vi "Demo_OK_COUNT.vi"(0 "Refnum in":T2, 1 "Station":string, 3 "Shift":i32, 5 "MAX BREAKDOWN ID":i32, 7 "PRODUCTION COUNT":i32, 9 "TABLE NAME":string, 11 "error in (no error)":errorcluster, 12 "Product Code for OK":string) -> (4 "Refnum out":T2, 6 "PROD COUNT":i32, 15 "error out":errorcluster)   [LabVIEW 2017]
uses:
  <vilib>/addons/database/Connection.llb/Conn ObjectReference.ctl
  <vilib>/addons/database/NI_Database_API.lvlib
  <userlib>/_OpenG.lib/comparison/comparison.llb/I32 Changed__ogtk.vi
panel:
  out "output":T1
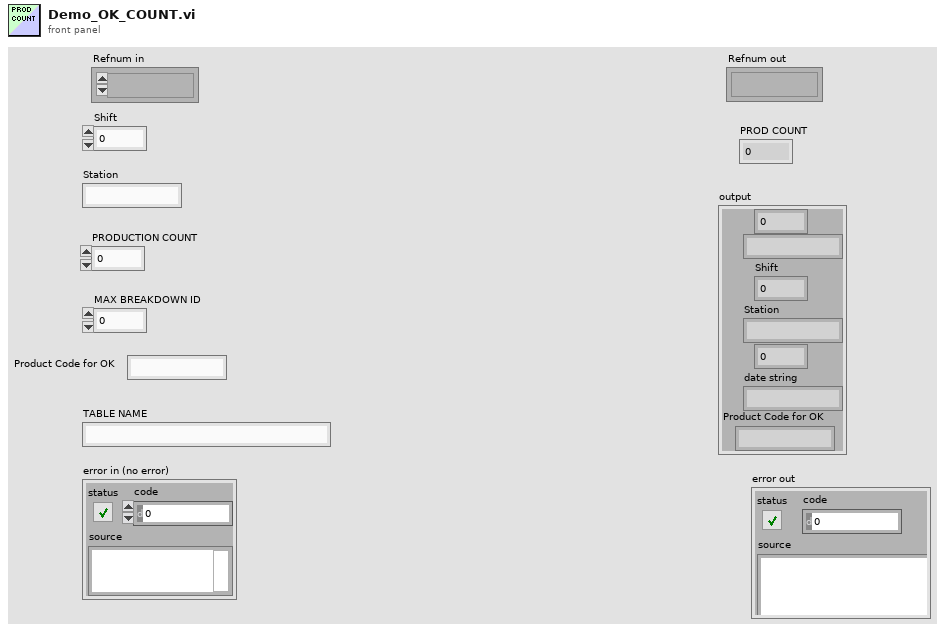
[diagram p1: front panel]
types:
  T1 = cluster{i32, string, "Shift":i32, "Station":string, i32, "date string":string, "Product Code for OK":string}
  T2 = typedef "NI_Database_API.lvlib/Conn ObjectReference.ctl" = refnum<k1>
  T3 = typedef "LVDateTimeRec.ctl" = cluster{"fractional second":dbl, "second":i32, "minute":i32, "hour":i32, "day of month":i32, "month":i32, "year":i32, "day of week":i32, "day of year":i32, "DST":i32}
  T4 = cluster{i32, "date/time string":string, "Shift":i32, "Station":string, i32, "Date String":string, "Product Code for OK":string}
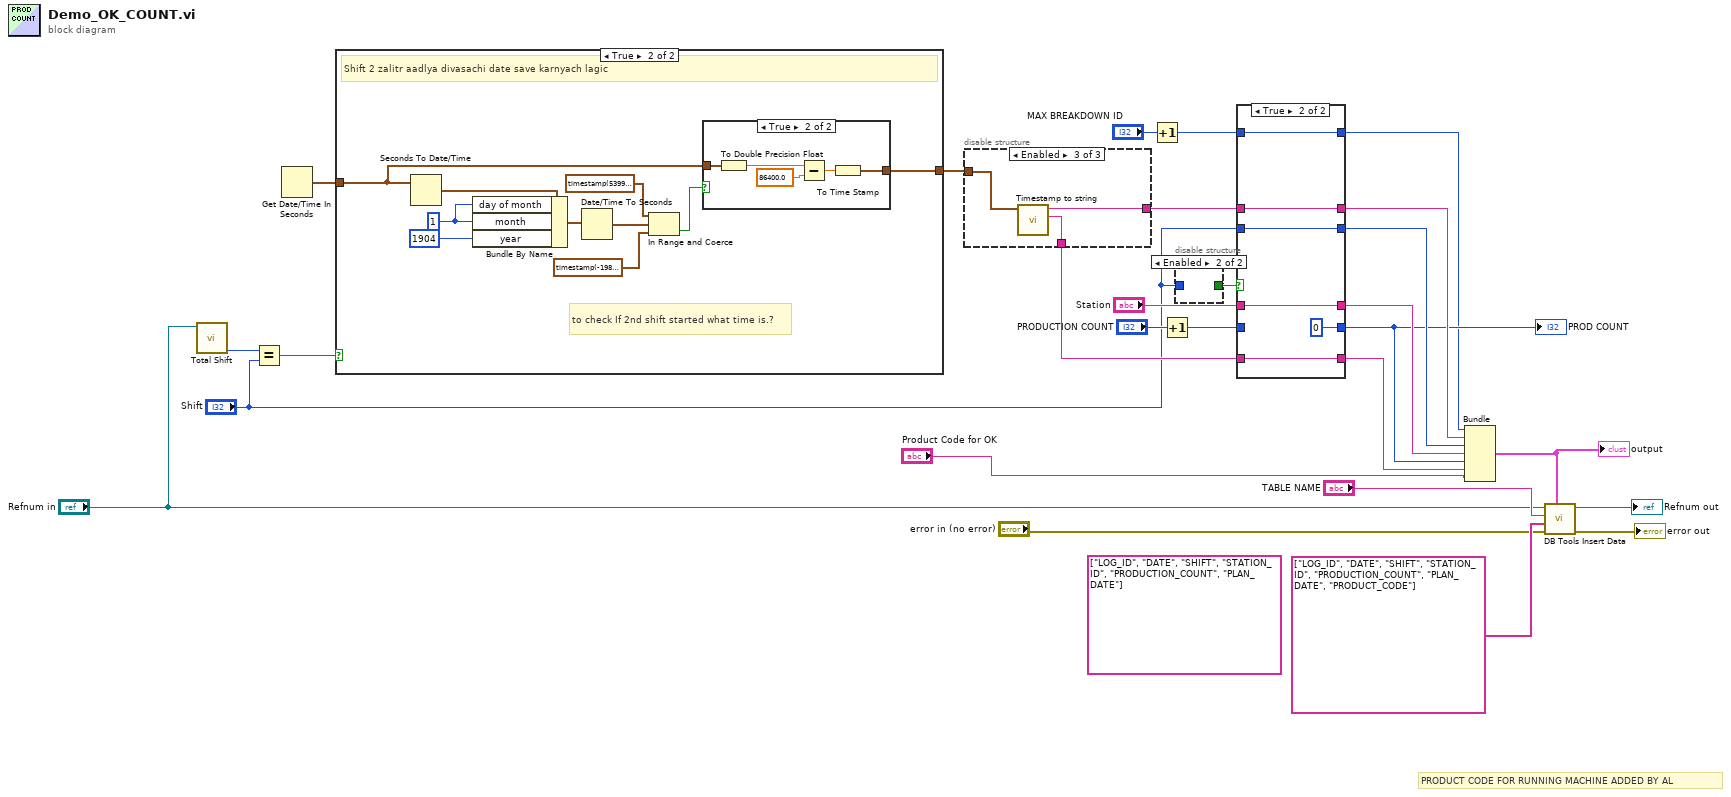
[diagram p0: block diagram]
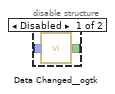
[diagram p2: hidden frame]
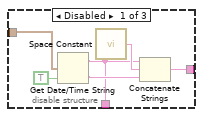
[diagram p3: hidden frame]
diagram:
  (unwired) string[] ["LOG_ID", "DATE", "SHIFT", "STATION_ID", "PRODUCTION_COUNT", "PLAN_DATE"] ("columns")
  # "PRODUCT CODE FOR RUNNING MACHINE ADDED BY AL"
  n1 = call "Total Shift.vi"("connection reference"="Refnum in") -> ("Total Shifts"=w6:i32)  [unwired: 9 in, 1 out]
  n2 = Equal?(x=w6, y="Shift") -> (x = y?=w7:bool)
  n3 = Get Date/Time In Seconds() -> (seconds since 1Jan1904=w4:timestamp)
  n4 = case shown="True" w7 {
    tunnel: w4 -> [w28 w29]
    tunnel: [w28 w30] -> w3
    frame False {
    }
    frame True {
      w35 = 1 ("day of month")
      # "to check If 2nd shift started what time is.?"
      # "Shift 2 zalitr aadlya divasachi date save karnyach lagic"
      n5 = Seconds To Date/Time(time stamp (now)=w29) -> (date time rec=w36:T3)  [unwired: 1 in]
      n6 = Bundle By Name(cluster=w36, "day of month"=w35, "month"=w35, "year"=1904) -> (w38:T3)
      n7 = Date/Time To Seconds(2:w38) -> (0:w34:timestamp)  [unwired: 1 in]
      n8 = In Range and Coerce(upper limit=timestamp(5399.999 s since 1904-01-01), x=w34, lower limit=timestamp(-19800 s since 1904-01-01)) -> (In Range?=w31:bool)  [unwired: 1 out]
      n9 = case shown="True" w31 {
        tunnel: [w39 w41] -> w30
        tunnel: w29 -> [w39 w40]
        frame False {
        }
        frame True {
          n10 = To Double Precision Float(number=w40) -> (double precision float=w44:dbl)
          n11 = Subtract(x=w44, y=86400.0) -> (x-y=w42:dbl)
          n12 = To Time Stamp(1:w42) -> (0:w41:timestamp)
        }
      }
    }
  }
  n13 = disable-structure shown="Enabled" {
    disable-tunnel: [w48 w51 w53] -> w19
    disable-tunnel: [w46 w51 w52] -> w9
    disable-tunnel: w3 -> [w45 w51 w54]
    frame Disabled {
      n14 = Get Date/Time String(seconds (now)=w45, want seconds? (F)=TRUE) -> (date string=w46:string, time string=w49:string)  [unwired: 1 in]
      n15 = call <vilib>:"Space Constant.vi"() -> ("String"=w50:string)
      n16 = Concatenate Strings(w46, w50, w49) -> (w48:string)
    }
    frame Disabled {
    }
    frame Enabled {
      n17 = call "Timestamp to string.vi"("time stamp"=w54) -> ("Date String"=w52:string, "date/time string"=w53:string)  [unwired: 8 in, 1 out]
    }
  }
  n18 = Increment(x="MAX BREAKDOWN ID") -> (x+1=w21:i32)
  n19 = Increment(x="PRODUCTION COUNT") -> (x+1=w14:i32)
  n20 = disable-structure shown="Enabled" {
    disable-tunnel: [w56 _] -> w22
    disable-tunnel: "Shift" -> [w55 _]
    frame Disabled {
      n21 = call-poly <userlib>:"Data Changed__ogtk.vi"("I32"=w55) -> ("Changed"=w56:bool)
    }
    frame Enabled {
    }
  }
  n22 = case shown="True" w22 {
    tunnel: [w62 w68] -> w11
    tunnel: w21 -> [w62 w68]
    tunnel: [w61 w67] -> w20
    tunnel: w19 -> [w61 w67]
    tunnel: [w60 w66] -> w18
    tunnel: "Shift" -> [w60 w66]
    tunnel: [w59 w65] -> w17
    tunnel: "Station" -> [w59 w65]
    tunnel: [w58 0] -> w13
    tunnel: w14 -> [w58 _]
    tunnel: [w57 w63] -> w10
    tunnel: w9 -> [w57 w63]
    frame False {
    }
    frame True {
    }
  }
  "PROD COUNT" <- w13
  n23 = Bundle(w11, "date/time string"=w20, "Shift"=w18, "Station"=w17, w13, "Date String"=w10, "Product Code for OK"="Product Code for OK") -> (w2:T4)  [unwired: 1 in]
  "output" <- w2
  n24 = call <vilib>:"DB Tools Insert Data.vi"("data"=w2, "error in (no error)"="error in (no error)", "columns"=string[] ["LOG_ID", "DATE", "SHIFT", "STATION_ID", "PRODUCTION_COUNT", "PLAN_DATE", "PRODUCT_CODE"], "table"="TABLE NAME", "connection reference"="Refnum in") -> ("error out"=→"error out":errorcluster, "connection reference out"=→"Refnum out":T2)  [unwired: 5 in]
